vi "UpdateSettings.ROIarray.vi"(8 "error in (no error)":errorcluster, 9 "ElementToUpdate":string, 10 "value":u16, 11 "ROI in":T1) -> (0 "error out":errorcluster, 3 "ROI out":T1)   [LabVIEW 2013, in "Photometrics_CH-250_Cam.lvclass"]
uses:
  Photometrics_CH-250_Cam.lvclass
  Point Grey Camera/subVis/ROI_TypDef.ctl
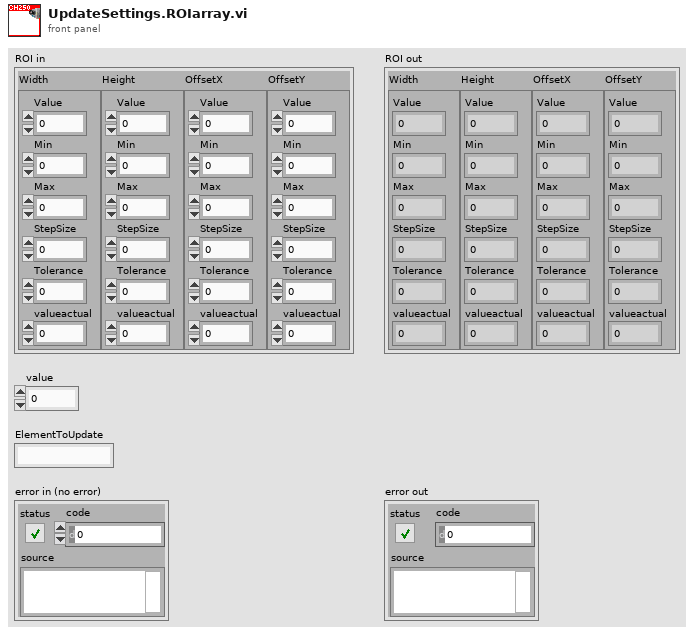
[diagram p1: front panel]
types:
  T1 = typedef "ROI_TypDef.ctl" = cluster{"Width":cluster{"Value":dbl, "Min":dbl, "Max":dbl, "StepSize":dbl, "Tolerance":dbl, "valueactual":dbl}, "Height":cluster{"Value":dbl, "Min":dbl, "Max":dbl, "StepSize":dbl, "Tolerance":dbl, "valueactual":dbl}, "OffsetX":cluster{"Value":dbl, "Min":dbl, "Max":dbl, "StepSize":dbl, "Tolerance":dbl, "valueactual":dbl}, "OffsetY":cluster{"Value":dbl, "Min":dbl, "Max":dbl, "StepSize":dbl, "Tolerance":dbl, "valueactual":dbl}}
  T2 = cluster{"Value":dbl, "Min":dbl, "Max":dbl, "StepSize":dbl, "Tolerance":dbl, "valueactual":dbl}
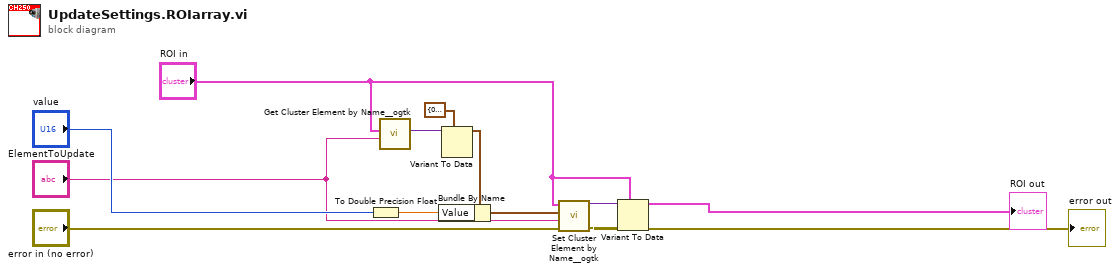
[diagram p0: block diagram]
diagram:
  n1 = To Double Precision Float(number="value") -> (double precision float=w12:dbl)
  n2 = call <userlib>:"Get Cluster Element by Name__ogtk.vi"("Element Name"="ElementToUpdate", "Cluster"="ROI in") -> ("VElement"=w6:variant)  [unwired: 7 in, 2 out]
  n3 = Variant To Data(type=T2 {"Value"=0.0, "Min"=0.0, "Max"=0.0, "StepSize"=0.0, "Tolerance"=0.0, "valueactual"=0.0} ("OffsetY"), Variant=w6) -> (data=w8:T2)  [unwired: 1 in, 1 out]
  n4 = Bundle By Name(cluster=w8, "Value"=w12) -> (w9:T2)
  n5 = call <userlib>:"Set Cluster Element by Name__ogtk.vi"("error in (no error)"="error in (no error)", "Element Name (\"\": New Element Data Name)"="ElementToUpdate", "New Element Value"=w9, "Cluster"="ROI in") -> ("error out"=w3:errorcluster, "VCluster out"=w2:variant)  [unwired: 5 in, 1 out]
  n6 = Variant To Data(error in=w3, type="ROI in", Variant=w2) -> (data=→"ROI out":T1, error out=→"error out":errorcluster)
